vi "receiveAllTelemetry.vi"(8 "error in (no error)":errorcluster, 11 "FPGATelemetry in":refnum<class "FPGATelemetry.lvclass">) -> (0 "error out":errorcluster, 2 "Telemetry":u32[](array[numeric]), 3 "FPGATelemetry out":refnum<class "FPGATelemetry.lvclass">)   [LabVIEW 2015, in "FPGATelemetry.lvclass"]
uses:
  FPGATelemetry.lvclass
  FPGATelemetry.lvclass/FPGATelemetry.ctl
  <vilib>/Utility/error.llb/Error Cluster From Error Code.vi
  <vilib>/rvi/errors/niLvFpgaAdjustHostInterfaceError.vi
  <vilib>/rvi/interface/nirviMethod/nirviMethod.xnode
  <vilib>/FPGAPlugInAG/Dynamic/niLvFpga_WriteFifo_Dynamic.vi
  <vilib>/rvi/errors/niLvFpgaMergeErrorWithErrorCode.vi
  <vilib>/FPGAPlugInAG/Dynamic/niLvFpga_ReadFifo_Dynamic.vi
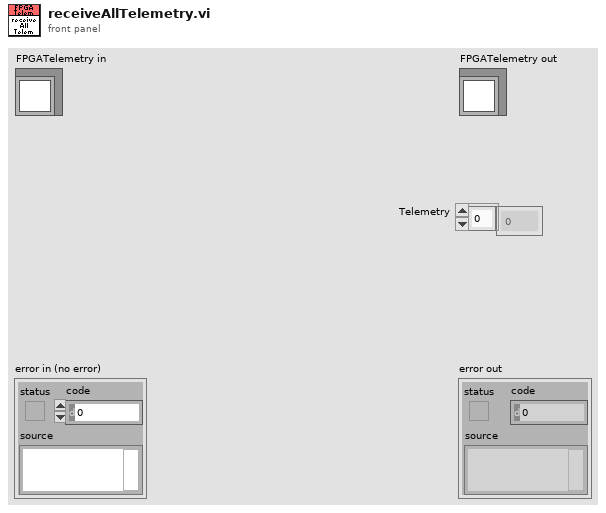
[diagram p1: front panel]
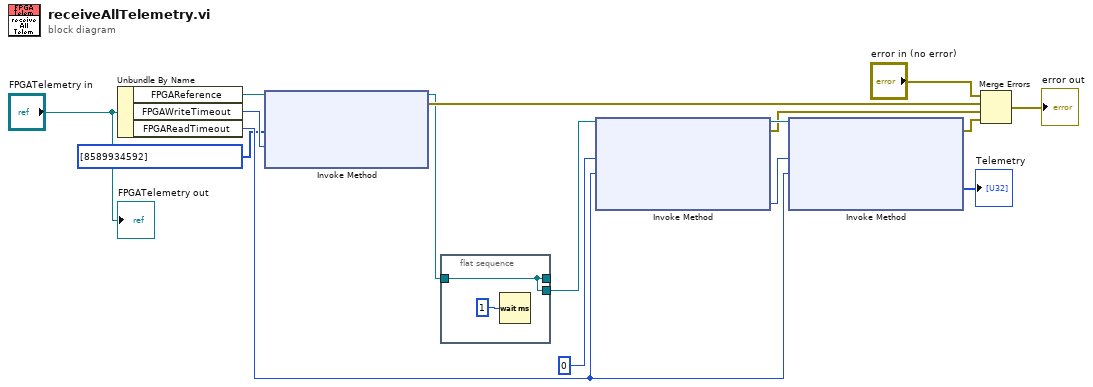
[diagram p0: block diagram]
diagram:
  n1 = Unbundle By Name("FPGATelemetry in") -> ("FPGAReference"=w16:refnum<k20>, "FPGAWriteTimeout"=w15:i32, "FPGAReadTimeout"=w12:i32)
  n2 = xnode "Invoke Method"("FPGA VI Reference In"=w16, "Data"=u64[] [8589934592], "Timeout (ms)"=w15) -> ("FPGA VI Reference Out"=w2:refnum<k20>, "error out"=w9:errorcluster)  [unwired: 1 in, 1 out]
  n3 = flat-sequence {
    tunnel: w2 -> [w17]
    tunnel: [w17] -> _
    tunnel: [w17] -> w1
    frame #0 {
      n4 = Wait (ms)(milliseconds to wait=u32 1) -> ()  [unwired: 1 out]
    }
  }
  n5 = xnode "Invoke Method"("FPGA VI Reference In"=w1, "Number of Elements"=u32 0, "Timeout (ms)"=w12) -> ("FPGA VI Reference Out"=w14:refnum<k20>, "error out"=w8:errorcluster, "Elements Remaining"=w11:u32)  [unwired: 1 in, 1 out]
  n6 = xnode "Invoke Method"("FPGA VI Reference In"=w14, "Number of Elements"=w11, "Timeout (ms)"=w12) -> ("error out"=w7:errorcluster, "Data"=→"Telemetry":u32[])  [unwired: 1 in, 2 out]
  n7 = Merge Errors("error in (no error)", w9, w8, w7) -> (→"error out":errorcluster)
  "FPGATelemetry out" <- "FPGATelemetry in"
